vi "read-lecory-xs.vi"() -> (0 "C2 data":cluster{dbl[], dbl[]})   [LabVIEW 2018]
panel:
  out "XY图":cluster{dbl[], dbl[]}[](graph)
  out "NumChannels":i32
  out "DeviceModel":string
  out "ConnectionType":string
  out "SetRemoteLocal":bool
  out "MakeConnection":bool
  in  "ActiveDSO":refnum<k7>(container)
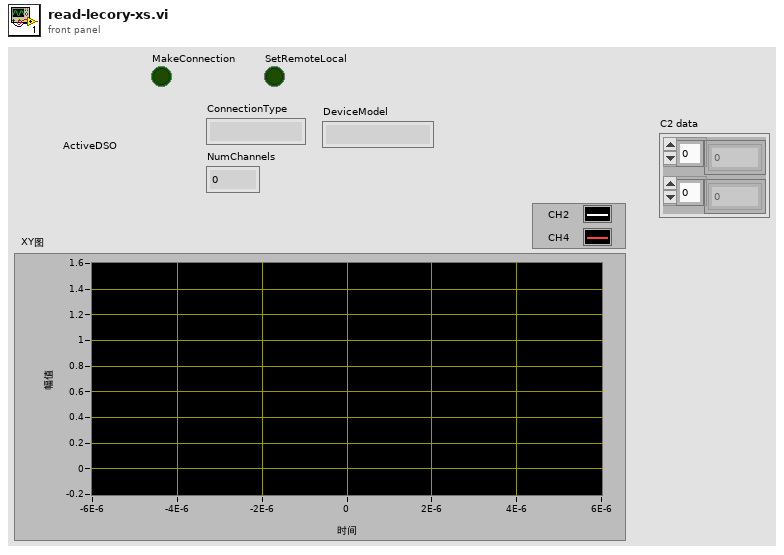
[diagram p1: front panel]
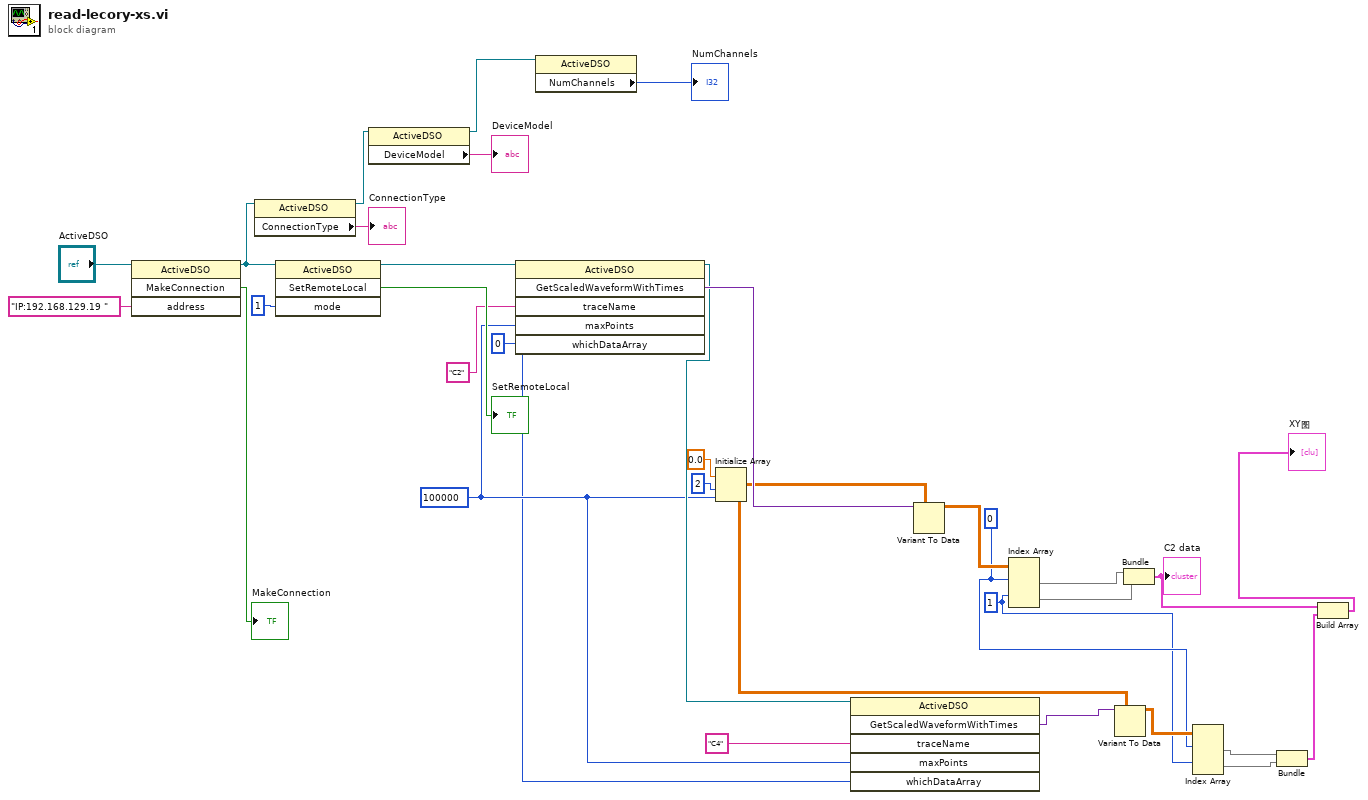
[diagram p0: block diagram]
diagram:
  w8 = 1 ("索引 (行)")
  w9 = 0 ("索引 (行)")
  w13 = i16 0 ("whichDataArray")
  w14 = 100000 ("maxPoints")
  n1 = invoke class="ActiveDSO" method="MakeConnection"(reference="ActiveDSO", "address"="IP:192.168.129.19 ") -> (reference out=w29:refnum<k7>, "MakeConnection"=→"MakeConnection":bool)  [unwired: 2 in, 2 out]
  n2 = property class="ActiveDSO"(reference=w29) -> (reference out=w27:refnum<k7>, "ConnectionType"=→"ConnectionType":string)  [unwired: 1 in, 1 out]
  n3 = invoke class="ActiveDSO" method="SetRemoteLocal"(reference=w29, "mode"=1) -> (reference out=w23:refnum<k7>, "SetRemoteLocal"=→"SetRemoteLocal":bool)  [unwired: 2 in, 2 out]
  n4 = property class="ActiveDSO"(reference=w27) -> (reference out=w25:refnum<k7>, "DeviceModel"=→"DeviceModel":string)  [unwired: 1 in, 1 out]
  n5 = invoke class="ActiveDSO" method="GetScaledWaveformWithTimes"(reference=w23, "traceName"="C2", "maxPoints"=w14, "whichDataArray"=w13) -> (reference out=w16:refnum<k7>, "GetScaledWaveformWithTimes"=w21:variant)  [unwired: 2 in, 4 out]
  n6 = property class="ActiveDSO"(reference=w25) -> ("NumChannels"=→"NumChannels":i32)  [unwired: 1 in, 2 out]
  n7 = Initialize Array(0.0 ("元素"), 2 ("维数大小"), w14) -> (w11:dbl[][])
  n8 = invoke class="ActiveDSO" method="GetScaledWaveformWithTimes"(reference=w16, "traceName"="C4", "maxPoints"=w14, "whichDataArray"=w13) -> ("GetScaledWaveformWithTimes"=w12:variant)  [unwired: 2 in, 5 out]
  n9 = Variant To Data(type=w11, Variant=w21) -> (data=w18:dbl[][])  [unwired: 1 in, 1 out]
  n10 = Index Array(array=w18, index (row) #1=w9, index (row) #2=w8) -> (element #1=w7:dbl[], element #2=w6:dbl[])  [unwired: 2 in]
  n11 = Variant To Data(type=w11, Variant=w12) -> (data=w10:dbl[][])  [unwired: 1 in, 1 out]
  n12 = Bundle(w7, w6) -> (w3:cluster{dbl[], dbl[]})  [unwired: 1 in]
  "C2 data" <- w3
  n13 = Index Array(array=w10, index (row) #1=w9, index (row) #2=w8) -> (element #1=w5:dbl[], element #2=w4:dbl[])  [unwired: 2 in]
  n14 = Bundle(w5, w4) -> (w2:cluster{dbl[], dbl[]})  [unwired: 1 in]
  n15 = Build Array(w3, w2) -> (→"XY图":cluster{dbl[], dbl[]}[])
